vi "Deserialise content.vi"(8 "error in (no error)":errorcluster, 10 "JSON String to decode":string, 11 "object in":refnum<class "execute_input Message.lvclass">) -> (0 "error out":errorcluster, 3 "object out":refnum<class "execute_input Message.lvclass">)   [LabVIEW 2018, in "ClientMessaging.lvlib" / "execute_input Message.lvclass"]
doc: "Convert content dictionary to class private data"
uses:
  execute_input Message.lvclass
  6515b34e-0c9a-446c-91af-f820618fdb14.vi
  59efa82c-bf54-48df-876a-8c19a0f95466.vi
  Base Classes/Message Class/Message Class.lvclass
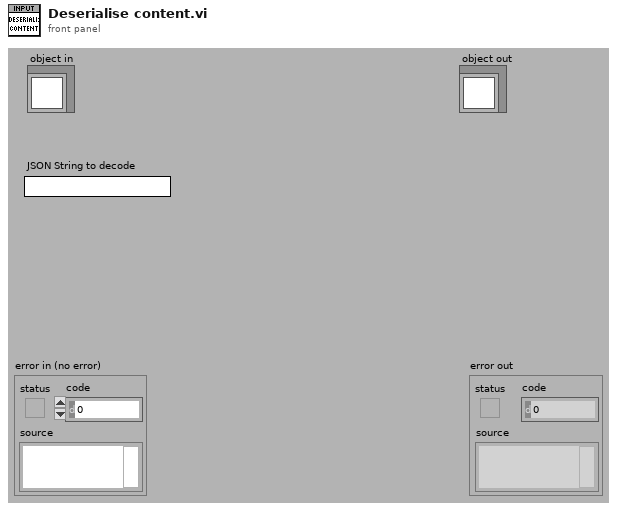
[diagram p1: front panel]
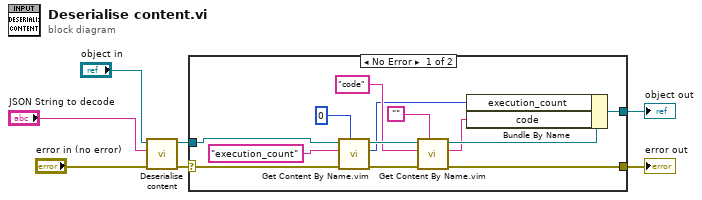
[diagram p0: block diagram]
diagram:
  n1 = call-parent "Deserialise content.vi"("error in (no error)"="error in (no error)", "JSON String to decode"="JSON String to decode", "object in"="object in") -> ("error out"=w1:errorcluster, "object out"=w4:refnum<class "execute_input Message.lvclass">)  [unwired: 7 in]
  n2 = case shown="No Error" w1 {
    selector: w1 -> [w9 w22]
    tunnel: [w8 w22] -> w7
    tunnel: [w12 w21] -> w5
    tunnel: w4 -> [w20 w21]
    frame No Error {
      n3 = call "Get Content By Name.vim"("Type of content"=0, "error in (no error)"=w9, "Name of Content Item"="execution_count", "Message In"=w20) -> ("error out"=w16:errorcluster, "Data Out"=w10:i32, "Message Out"=w17:refnum<class "execute_input Message.lvclass">)  [unwired: 5 in]
      n4 = call "Get Content By Name.vim"("Type of content"="", "error in (no error)"=w16, "Name of Content Item"="code", "Message In"=w17) -> ("error out"=w8:errorcluster, "Data Out"=w11:string, "Message Out"=w13:refnum<class "execute_input Message.lvclass">)  [unwired: 5 in]
      n5 = Bundle By Name(cluster=w13, "execution_count"=w10, "code"=w11) -> (w12:refnum<class "execute_input Message.lvclass">)
    }
    frame Error {
    }
  }
  "error out" <- w7
  "object out" <- w5
